vi "FindColoredObject.vi"(6 "Color Range":T3={"Hue"={"Lower"=55, "Upper"=93}, "Sat"={"Lower"=41, "Upper"=255}, " Luma"={"Lower"=99, "Upper"=255}}, 8 "Decimate by":cluster{"H":i32, "V":i32}={"H"=3, "V"=5}, 9 "Color Image In":T1) -> (0 "Area":i32, 1 "Particles":i32, 2 "Rectangle":T2, 3 "Mask Image":T1)   [LabVIEW 2011]
doc: "Given and image and a color range, return information about the largest object that matches the color description. Return values incllude the rectangle surrounding the object, the pixel area of the object, and the number of overall particles or objects that matched the color. Mask can be used with an image display to view what matches the color range. Be sure to right click and set the color palette of the display to Binary."
uses:
  <vilib>/vision/Image Controls.llb/IMAQ Image.ctl
  <vilib>/vision/NI_Vision_Development_Module.lvlib
panel:
  in  "HSL Debug":bool
  out "Find Time":u32
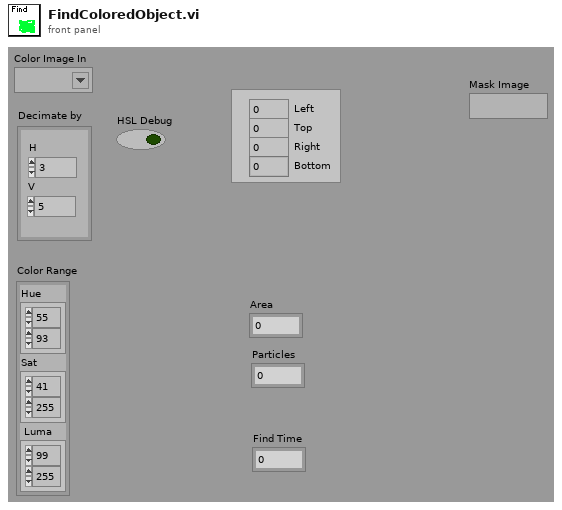
[diagram p1: front panel]
types:
  T1 = typedef "IMAQ Image.ctl" = refnum<image>
  T2 = cluster{"Left":i32, "Top":i32, "Right":i32, "Bottom":i32}
  T3 = cluster{"Hue":cluster{"Lower":i32, "Upper":i32}, "Sat":cluster{"Lower":i32, "Upper":i32}, " Luma":cluster{"Lower":i32, "Upper":i32}}
  T4 = typedef "Image Type" = u32
  T5 = cluster{"New Image":T1, "New Image":T1, "New Image":T1}
  T6 = cluster{"Pixel Area":dbl, "Rectangle":cluster{"Left":i32, "Top":i32, "Right":i32, "Bottom":i32}}[]
  T7 = cluster{"Pixel Area":dbl, "Rectangle":cluster{"Left":i32, "Top":i32, "Right":i32, "Bottom":i32}}
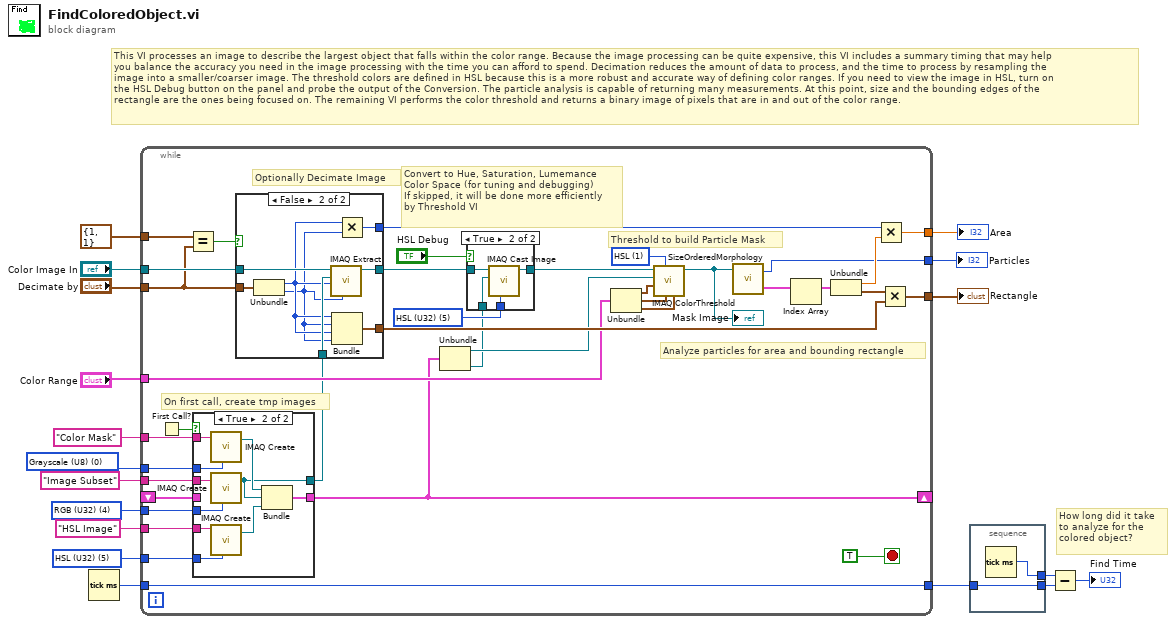
[diagram p0: block diagram]
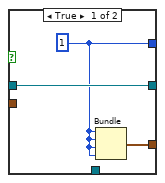
[diagram p3: hidden frame]
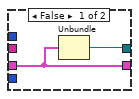
[diagram p4: hidden frame]
diagram:
  w2 = T4 5 items=["Grayscale (U8)", "Grayscale (I16)", "Grayscale (SGL)", "Complex (CSG)", "RGB (U32)", "HSL (U32)", "RGB (U64)"] ("Image Type")
  w11 = T4 0 items=["Grayscale (U8)", "Grayscale (I16)", "Grayscale (SGL)", "Complex (CSG)", "RGB (U32)", "HSL (U32)", "RGB (U64)"] ("Image Type")
  w16 = T4 4 items=["Grayscale (U8)", "Grayscale (I16)", "Grayscale (SGL)", "Complex (CSG)", "RGB (U32)", "HSL (U32)", "RGB (U64)"] ("Image Type")
  # "How long did it take\nto analyze for the\ncolored object?"
  # "This VI processes an image to describe the largest object that falls within the color range. Because the image processing can be quite expensive, this VI includes a summary timing that may help\nyou balance the accuracy you need in the image processing with the time you can afford to spend. Decimation reduces the amount of data to process, and the time to process by resampling the\nimage into a smaller/coarser image. The threshold colors are defined in HSL because this is a more robust and accurate way of defining color ranges. If you need to view the image in HSL, turn on\nthe HSL Debug button on the panel and probe the output of the Conversion. The particle analysis is capable of returning many measurements. At this point, size and the bounding edges of the\nrectangle are the ones being focused on. The remaining VI performs the color threshold and returns a binary image of pixels that are in and out of the color range."
  n1 = Tick Count (ms)() -> (millisecond timer value=w18:u32)
  n2 = while {
    tunnel: "Color Image In" -> [w54]
    tunnel: [w27] -> w7
    tunnel: w18 -> [w44]
    shift-right: [w39] -> _
    shift-left: _ -> [w52]
    tunnel: "Image Subset" ("Image Name") -> [w51]
    tunnel: w16 -> [w50]
    tunnel: [w44] -> w14
    tunnel: [w45] -> w6
    tunnel: "Color Range" -> [w42]
    tunnel: [w43] -> w5
    tunnel: w11 -> [w41]
    tunnel: "Color Mask" ("Image Name") -> [w40]
    tunnel: "Decimate by" -> [w34]
    tunnel: cluster{"H":i32, "V":i32} {"H"=1, "V"=1} ("x") -> [w26]
    tunnel: w2 -> [w21]
    tunnel: "HSL Image" ("Image Name") -> [w20]
    stop <- TRUE stop-if-true
    w49 = u16 1 items=["RGB", "HSL", "HSV", "HSI"] ("Color Mode")
    w48 = T4 5 items=["Grayscale (U8)", "Grayscale (I16)", "Grayscale (SGL)", "Complex (CSG)", "RGB (U32)", "HSL (U32)", "RGB (U64)"] ("Image Type")
    # "On first call, create tmp images"
    # "Analyze particles for area and bounding rectangle"
    # "Convert to Hue, Saturation, Lumemance\nColor Space (for tuning and debugging)\nIf skipped, it will be done more efficiently\nby Threshold VI"
    # "Optionally Decimate Image"
    # "Threshold to build Particle Mask"
    n3 = First Call?() -> (First Call?: T/F=w53:bool)
    n4 = Equal?(x=w26, y=w34) -> (x = y?=w33:bool)
    n5 = case shown="True" w53 {
      tunnel: w51 -> [_ w83]
      tunnel: w50 -> [_ w82]
      tunnel: w52 -> [w73 _]
      tunnel: [w73 w80] -> w39
      tunnel: w41 -> [_ w79]
      tunnel: w40 -> [_ w78]
      tunnel: [w72 w77] -> w32
      tunnel: w21 -> [_ w76]
      tunnel: w20 -> [_ w75]
      frame False {
        n6 = Unbundle(w73) -> ("New Image"=w72:T1)  [unwired: 2 out]
      }
      frame True {
        n7 = call "IMAQ Create"("Image Name"=w78, "Image Type"=w79) -> ("New Image"=w81:T1)  [unwired: 2 in, 2 out]
        n8 = call "IMAQ Create"("Image Name"=w83, "Image Type"=w82) -> ("New Image"=w77:T1)  [unwired: 2 in, 2 out]
        n9 = call "IMAQ Create"("Image Name"=w75, "Image Type"=w76) -> ("New Image"=w74:T1)  [unwired: 2 in, 2 out]
        n10 = Bundle("New Image"=w81, "New Image"=w77, "New Image"=w74) -> (w80:T5)  [unwired: 1 out]
      }
    }
    n11 = case shown="False" w33 {
      tunnel: w54 -> [w63 w71]
      tunnel: [w63 w69] -> w23
      tunnel: w32 -> [_ w70]
      tunnel: [w62 w68] -> w46
      tunnel: w34 -> [_ w67]
      tunnel: [w61 w66] -> w47
      frame True {
        w62 = 1
        n12 = Bundle(w62, w62, w62, w62) -> (w61:cluster{i32, i32, i32, i32})  [unwired: 1 out]
      }
      frame False {
        n13 = Unbundle(w67) -> ("H"=w65:i32, "V"=w64:i32)
        n14 = call "IMAQ Extract"("Y Step Size"=w64, "X Step Size"=w65, "Image Dst"=w70, "Image Src"=w71) -> ("Image Dst Out"=w69:T1)  [unwired: 2 in, 5 out]
        n15 = Bundle("H"=w65, "V"=w64, "H"=w65, "V"=w64) -> (w66:cluster{"H":i32, "V":i32, "H":i32, "V":i32})  [unwired: 1 out]
        n16 = Multiply(x=w65, y=w64) -> (x*y=w68:i32)
      }
    }
    n17 = Unbundle(w39) -> ("New Image"=w38:T1, "New Image"=w19:T1)  [unwired: 1 out]
    n18 = case shown="True" "HSL Debug" {
      tunnel: w48 -> [_ w60]
      tunnel: w23 -> [w56 w59]
      tunnel: [w56 w58] -> w22
      tunnel: w19 -> [_ w57]
      frame False {
      }
      frame True {
        n19 = call "IMAQ Cast Image"("Image Type"=w60, "Image Dst"=w57, "Image Src"=w59) -> ("Image Dst Out"=w58:T1)  [unwired: 3 in, 5 out]
      }
    }
    n20 = Unbundle(w42) -> ("Hue"=w35:cluster{"Lower":i32, "Upper":i32}, "Sat"=w37:cluster{"Lower":i32, "Upper":i32}, "Luma"=w36:cluster{"Lower":i32, "Upper":i32})
    n21 = call "IMAQ ColorThreshold"("Blue or Luma or Val or Inten Range"=w36, "Green or Sat Range"=w37, "Color Mode"=w49, "Red or Hue Range"=w35, "Image Dst"=w38, "Image Src"=w22) -> ("Image Dst Out"=w25:T1)  [unwired: 2 in, 3 out]
    "Mask Image" <- w25
    n22 = call "SizeOrderedMorphology.vi"("Image Dst Out"=w25) -> (0:"Particles"=w31:T6, 1:"Particles"=w27:i32)  [unwired: 1 in]
    n23 = Index Array(array=w31) -> (element=w30:T7)  [unwired: 1 in]
    n24 = Unbundle(w30) -> ("Pixel Area"=w29:dbl, "Rectangle"=w28:T2)
    n25 = Multiply(x=w46, y=w29) -> (x*y=w45:dbl)
    n26 = Multiply(x=w28, y=w47) -> (x*y=w43:cluster{i32, i32, i32, i32})
  }
  "Area" <- w6
  "Particles" <- w7
  "Rectangle" <- w5
  n27 = stacked-sequence {
    tunnel: [w85] -> w15
    tunnel: w14 -> [w85]
    tunnel: [w84] -> w13
    frame #0 {
      n28 = Tick Count (ms)() -> (millisecond timer value=w84:u32)
    }
  }
  n29 = Subtract(x=w13, y=w15) -> (x-y=→"Find Time":u32)
